vi "ExCircularBufferTifFileHeader.vi"() -> ()   [LabVIEW 2010]
panel:
  in  "Trigger Edge":u32(ring)=1 items=["", "Positive (leading) edge", "Negative (falling) Edge"]
  in  "Trigger/Timing Mode":u32(ring)=1 items=["N/A", "FreeRun/Timed", "Single Trigger (PM only)", "Ext Sync/Strobed", "Bulb (PM only)", "Variable (PM only)", "Flash Mode (PM only)"]
  in  "Temperature":dbl=-10.0 format="%.2f"
  in  "Exposure":dbl min=0.0 step=0.001 format="%.3f"
  in  "stop":bool
  in  "Store":bool
  out "error out":errorcluster
  in  "error in (no error)":errorcluster
  # "ExCircularBufferSpeFileHeader:\nThis example collects a full image using circular buffers.  It will save experiment\ninformation in the Spe file header.\nNote: not all cameras support circular buffers."
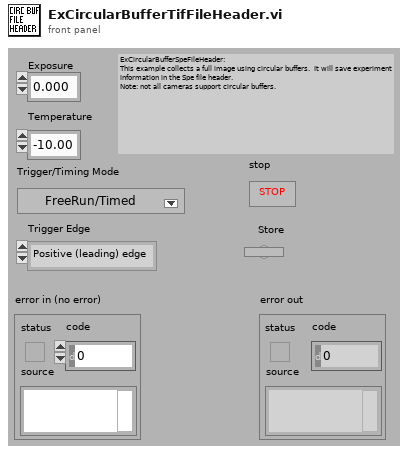
[diagram p1: front panel]
types:
  T1 = cluster{"acquire Mode\nSync-Focus \nNote: not all \ncameras support \nthis mode":i32, "Exposure":dbl, "Number of frames":i32, "Software Accumulations":i32}
  T2 = cluster{"Camera Handle":u32, "Pulser Handle":u32, "File Handle":u32, "Display Handle":u32, "Image Handle":u32}
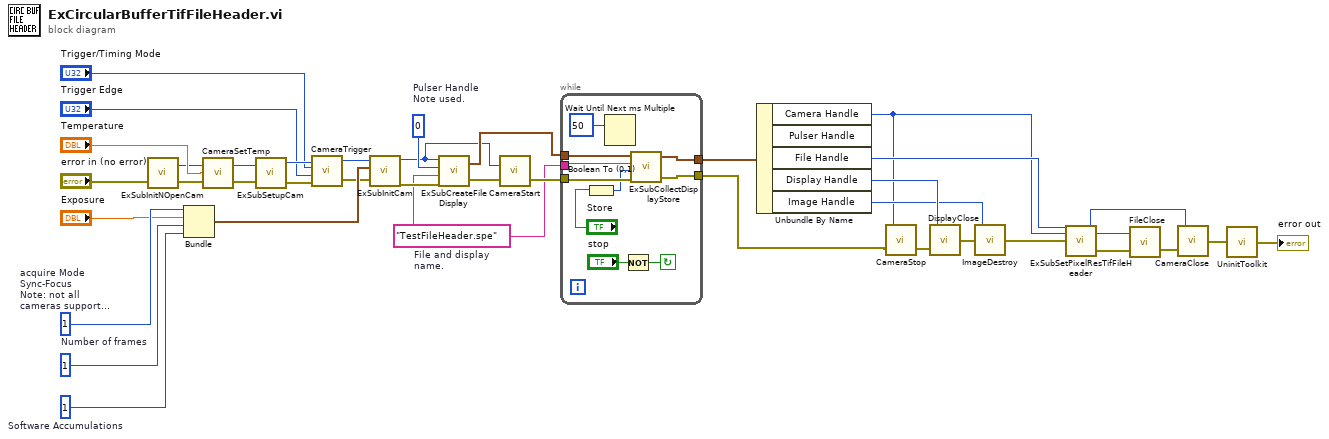
[diagram p0: block diagram]
diagram:
  w32 = 0  # Pulser Handle Note used.
  w38 = 1  # Number of frames
  w39 = 1  # acquire Mode Sync-Focus  Note: not all  cameras support  this mode
  w37 = 1  # Software Accumulations
  w12 = "TestFileHeader.spe"  # File and display  name.
  n1 = call "ExSubInitNOpenCam.vi"("error in (no error)"="error in (no error)") -> ("Camera Handle"=w21:u32, "error out"=w22:errorcluster)
  n2 = Bundle("acquire Mode\nSync-Focus \nNote: not all \ncameras support \nthis mode"=w39, "Exposure"="Exposure", "Number of frames"=w38, "Software Accumulations"=w37) -> (w34:T1)  [unwired: 1 in]
  n3 = call <userlib>:"CameraSetTemp.vi"("error in (no error)"=w22, "Temperature"="Temperature", "Camera Handle"=w21) -> ("error out"=w20:errorcluster, "Camera Handle"=w19:u32)
  n4 = call "ExSubSetupCam.vi"("error in (no error)"=w20, "Camera Handle"=w19) -> ("error out"=w26:errorcluster, "Camera Handle"=w28:u32)
  n5 = call <userlib>:"CameraTrigger.vi"("error in"=w26, "Trigger Edge"="Trigger Edge", "Timing Mode"="Trigger/Timing Mode", "Camera Handle"=w28) -> ("error out"=w29:errorcluster, "Camera Handle"=w27:u32)
  n6 = call "ExSubInitCam.vi"("error in (no error)"=w29, "Camera Information"=w34, "Camera Handle"=w27) -> ("error out"=w33:errorcluster, "Camera Handle"=w30:u32)
  n7 = call "ExSubCreateFileDisplay.vi"("error in (no error)"=w33, "File and Display Name"=w12, "Pulser Handle"=w32, "Camera Handle"=w30) -> ("error out"=w24:errorcluster, "Handles Out"=w31:T2)
  n8 = call <userlib>:"CameraStart.vi"("error in"=w24, "Camera Handle"=w30) -> ("error out"=w25:errorcluster)  [unwired: 1 out]
  n9 = while {
    tunnel: w31 -> [w48]
    tunnel: w25 -> [w46]
    tunnel: w12 -> [w47]
    tunnel: [w44] -> w15
    tunnel: [w45] -> w16
    stop <- w42 continue-if-true
    n10 = Boolean To (0,1)(Boolean="Store") -> (0, 1=w40:i16)
    n11 = Wait Until Next ms Multiple(millisecond multiple=50) -> ()  [unwired: 1 out]
    n12 = Not(x="stop") -> (.not. x?=w42:bool)
    n13 = call "ExSubCollectDisplayStore.vi"("error in (no error)"=w46, "Store flag"=w40, "Display Title"=w47, "Handle Cluster"=w48) -> ("error out"=w44:errorcluster, "Handle Cluster Out"=w45:T2)  [unwired: 1 out]
  }
  n14 = Unbundle By Name(w16) -> ("Camera Handle"=w8:u32, "File Handle"=w10:u32, "Display Handle"=w14:u32, "Image Handle"=w13:u32)  [unwired: 1 out]
  n15 = call <userlib>:"CameraStop.vi"("error in"=w15, "Camera Handle"=w8) -> ("error out"=w7:errorcluster)  [unwired: 1 out]
  n16 = call <userlib>:"DisplayClose.vi"("error in"=w7, "Display Handle"=w14) -> ("error out"=w11:errorcluster)
  n17 = call <userlib>:"ImageDestroy.vi"("error in"=w11, "Data handle"=w13) -> ("error out"=w6:errorcluster)
  n18 = call "ExSubSetPixelResTifFileHeader.vi"("error in (no error)"=w6, "Camera Handle"=w8, "File Handle"=w10) -> ("error out"=w5:errorcluster, "Camera Handle"=w1:u32, "File Handle"=w9:u32)
  n19 = call <userlib>:"FileClose.vi"("error in"=w5, "File Handle"=w9) -> ("error out"=w4:errorcluster)
  n20 = call <userlib>:"CameraClose.vi"("error in"=w4, "Camera Handle"=w1) -> ("error out"=w3:errorcluster)
  n21 = call <userlib>:"UninitToolkit.vi"("error in"=w3) -> ("error out"=→"error out":errorcluster)
